vi "NanotecSMCPDDriver.set max velocity.vi"(0 "VISA resource name":refnum<visa-resource-name>, 1 "contollerID":i32=-1, 3 "maxVelocity [Hz]":i32, 5 "error in (no error)":errorcluster) -> (14 "VISA resource name out":refnum<visa-resource-name>, 15 "contollerID out":i32=-1, 19 "error out":errorcluster)   [LabVIEW 2014, in "NanotecSMCPDDriver.lvlib"]
doc: "Sets the maximum velocity (\"stop frequency\") that will be used for the trajectory of a movement."
uses:
  NanotecSMCPDDriver.lvlib
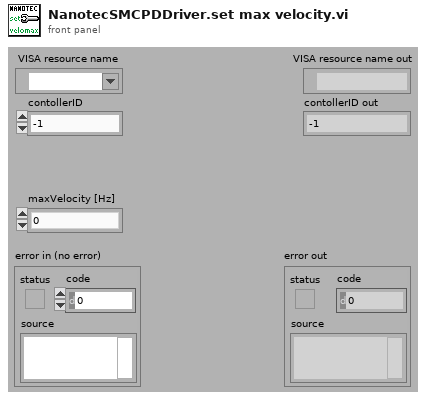
[diagram p1: front panel]
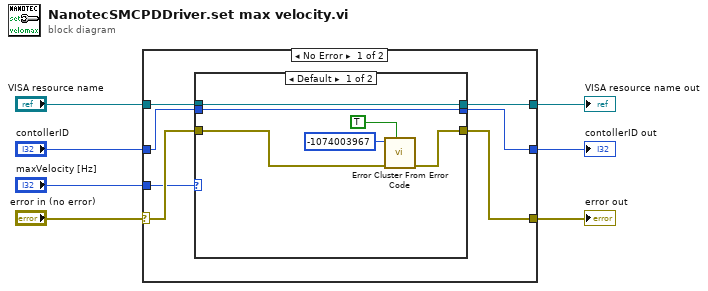
[diagram p0: block diagram]
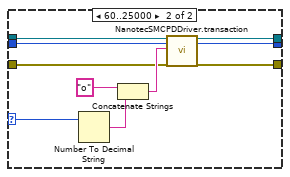
[diagram p2: hidden frame]
diagram:
  n1 = case shown="No Error" "error in (no error)" {
    selector: "error in (no error)" -> [w9 w31]
    tunnel: [w13 w33] -> w7
    tunnel: [w12 w31] -> w6
    tunnel: "VISA resource name" -> [w11 w33]
    tunnel: "contollerID" -> [w10 w32]
    tunnel: [w14 w32] -> w3
    tunnel: "maxVelocity [Hz]" -> [w8 _]
    frame No Error {
      n2 = case shown="Default" w8 {
        selector: w8 -> [_ w24]
        tunnel: [w16 w30] -> w14
        tunnel: [w17 w29] -> w13
        tunnel: [w20 w28] -> w12
        tunnel: w11 -> [w17 w23]
        tunnel: w10 -> [w16 w22]
        tunnel: w9 -> [w15 w21]
        frame Default {
          n3 = call <vilib>:"Error Cluster From Error Code.vi"("show call chain? (False)"=TRUE, "error in (no error)"=w15, "error code (0)"=-1074003967) -> ("error out"=w20:errorcluster)  [unwired: 6 in]
        }
        frame 60..25000 {
          n4 = Number To Decimal String(number=w24) -> (decimal integer string=w27:string)  [unwired: 1 in]
          n5 = Concatenate Strings("o" ("commandString"), w27) -> (w25:string)
          n6 = call "NanotecSMCPDDriver.transaction.vi"("VISAresource"=w23, "contollerID"=w22, "commandString"=w25, "error in (no error)"=w21) -> ("VISAresource out"=w29:refnum<visa-resource-name>, "contollerID out"=w30:i32, "error out"=w28:errorcluster)  [unwired: 10 in, 3 out]
        }
      }
    }
    frame Error {
    }
  }
  "VISA resource name out" <- w7
  "error out" <- w6
  "contollerID out" <- w3
